vi "Read Joystick 3.vi"   [LabVIEW 2011]
uses:
  Robot Global Data.vi
types:
  T1 = typedef "WPI_JoystickDevRef.ctl" = cluster{"Device":T2}
  T2 = typedef "WPI_JoystickDeviceEnum.ctl" = enum16{"USB 1", "USB 2", "USB 3", "USB 4", "Kinect 1", "Kinect 2"}
  T3 = typedef "WPI_JoystickButtonState.ctl" = cluster{"Button 1":bool, "Button 2":bool, "Button 3":bool, "Button 4":bool, "Button 5":bool, "Button 6":bool, "Button 7":bool, "Button 8":bool, "Button 9":bool, "Button 10":bool, "Button 11":bool, "Button 12":bool}
  T4 = cluster{"axis 1 (x)":dbl, "axis 2 (y)":dbl, "axis 3 (throttle)":dbl, "axis 4":dbl, "axis 5":dbl, "axis 6":dbl}
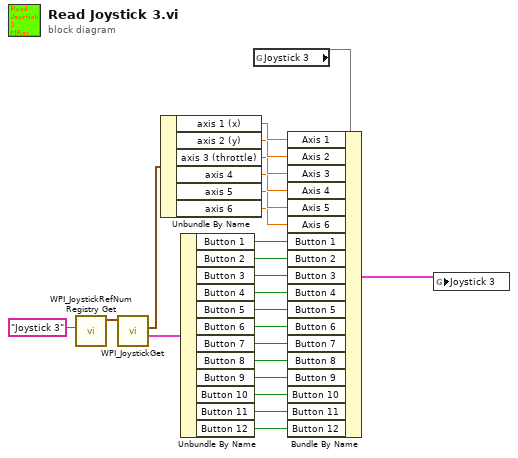
[diagram p0: block diagram]
diagram:
  n1 = call <vilib>:"WPI_JoystickRefNum Registry Get.vi"("refnum name"="Joystick 3") -> ("JoystickDevRef"=w24:T1)  [unwired: 9 in, 1 out]
  n2 = call <vilib>:"WPI_JoystickGet.vi"("JoystickDevRef"=w24) -> ("Buttons"=w22:T3, "Axes"=w23:T4)  [unwired: 4 in, 1 out]
  n3 = Unbundle By Name(w23) -> ("axis 1 (x)"=w21:dbl, "axis 2 (y)"=w20:dbl, "axis 3 (throttle)"=w19:dbl, "axis 4"=w18:dbl, "axis 5"=w17:dbl, "axis 6"=w16:dbl)
  n4 = Unbundle By Name(w22) -> ("Button 1"=w15:bool, "Button 2"=w14:bool, "Button 3"=w13:bool, "Button 4"=w12:bool, "Button 5"=w11:bool, "Button 6"=w10:bool, "Button 7"=w9:bool, "Button 8"=w8:bool, "Button 9"=w7:bool, "Button 10"=w6:bool, "Button 11"=w5:bool, "Button 12"=w4:bool)
  n5 = global read "Robot Global Data.vi" "Joystick 3"() -> (w2)
  n6 = Bundle By Name(cluster=w2, "Axis 1"=w21, "Axis 2"=w20, "Axis 3"=w19, "Axis 4"=w18, "Axis 5"=w17, "Axis 6"=w16, "Button 1"=w15, "Button 2"=w14, "Button 3"=w13, "Button 4"=w12, "Button 5"=w11, "Button 6"=w10, "Button 7"=w9, "Button 8"=w8, "Button 9"=w7, "Button 10"=w6, "Button 11"=w5, "Button 12"=w4) -> (w1:cluster{})
  n7 = global write "Robot Global Data.vi" "Joystick 3"(w1) -> ()
